vi "Subscribe.vi"(8 "error in (no error)":errorcluster, 10 "Subscription Request":refnum<class "SubscriptionRequest.lvclass">, 11 "IMediator In":refnum<class "IMediator.lvclass">) -> (0 "error out":errorcluster, 3 "IMediator Out":refnum<class "IMediator.lvclass">)   [LabVIEW 2018, in "MVA Framework.lvlib" / "IMediator.lvlib" / "IMediator.lvclass"]
doc: "抽象方法\n订阅"
uses:
  IMediator.lvclass
  SubscriptionRequest/SubscriptionRequest.lvclass
panel:
  # "Who wants it? (Unique Subscriber ID)\nWhat do they want? (Datum Name and Type)\nWhere/how do they want it sent? (Transport)\nWhen/under what conditions? (SubscriptionPolicy)"
  # "谁想要？（唯一订阅者ID）\n他们想要什么？（基准名称和类型）\n他们想把它寄到哪里/怎么寄？（运输）\n何时/在什么条件下？（订阅政策）"
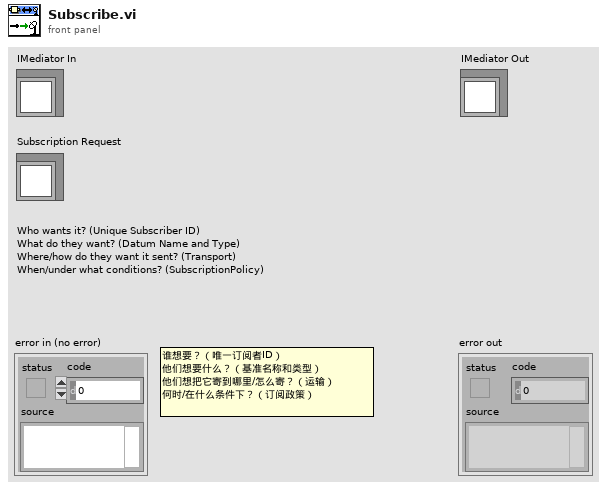
[diagram p1: front panel]
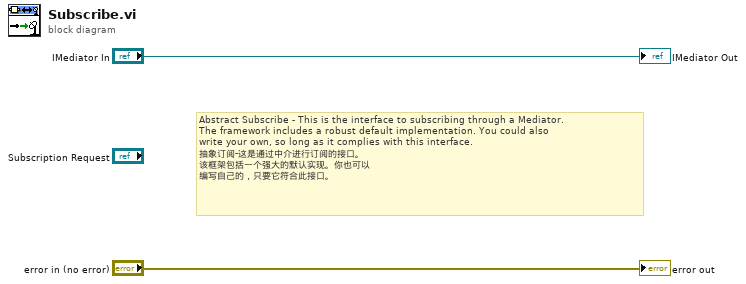
[diagram p0: block diagram]
diagram:
  # "Abstract Subscribe - This is the interface to subscribing through a Mediator.\nThe framework includes a robust default implementation. You could also\nwrite your own, so long as it complies with this interface.\n抽象订阅-这是通过中介进行订阅的接口。\n该框架包括一个强大的默认实现。你也可以\n编写自己的，只要它符合此接口。"
  "error out" <- "error in (no error)"
  "IMediator Out" <- "IMediator In"
